vi "Test U8 Logic.vi"() -> ()   [LabVIEW 2021]
uses:
  Source/Abs_Types/U8 Integer/Simple Read.vi
  Source/Constants/Support/U8/Const_U8.lvclass
  C:/TSA/LV_Abstract/Source/Abs_Types/U8 Integer/Abs_U8 Integer.lvclass
  C:/TSA/LV_Abstract/Source/Abs_Types/Integer/Abs_Integer.lvclass
  Source/Constants/Support/U8/U8.vi
  Source/Functions/Logic/Support/NOT/U8/Method.vi
  Source/Functions/Logic/Support/EXOR/U8/Method.vi
  Source/Functions/Logic/Support/EXNOR/U8/Method.vi
  Source/Functions/Logic/Support/NOR/U8/Method.vi
  Source/Functions/Logic/Support/OR/U8/Method.vi
  Source/Functions/Logic/Support/AND/U8/Method.vi
  Source/Abs_Types/U8 Integer/Abs_U8 Integer.lvclass
  C:/Program Files (x86)/National Instruments/LabVIEW 2021/vi.lib/TSA/Abstract Data Classes/Abs_Types/Numeric/Abs_Numeric.lvclass
  C:/Program Files (x86)/National Instruments/LabVIEW 2021/vi.lib/TSA/Abstract Data Classes/Abs_Types/Value/Abs_Value.lvclass
  C:/Program Files (x86)/National Instruments/LabVIEW 2021/vi.lib/TSA/Abstract Data Classes/Abs_Types/Type/Abs_Type.lvclass
  C:/TSA/LV_Abstract/Source/Constants/Support/U8/Const_U8.lvclass
  Source/Functions/Logic/Support/NOT/U8/NOT_U8.lvclass
  Source/Functions/Logic/Support/AND/U8/AND_U8.lvclass
  Source/Functions/Logic/Support/OR/U8/OR_U8.lvclass
  Source/Functions/Logic/Support/NOR/U8/NOR_U8.lvclass
  Source/Functions/Logic/Support/EXNOR/U8/EXNOR_U8.lvclass
  Source/Functions/Logic/Support/EXOR/U8/EXOR_U8.lvclass
panel:
  out "EXNOR":u8 format="%08b"
  out "NOR":u8 format="%08b"
  out "OR":u8 format="%08b"
  out "AND":u8 format="%08b"
  out "EXOR":u8 format="%08b"
  in  "Numeric 2":u8 format="%08b"
  in  "Numeric":u8 format="%08b"
  out "Not":u8 format="%08b"
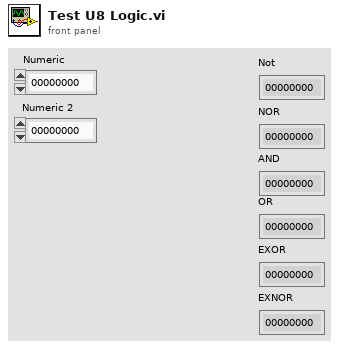
[diagram p1: front panel]
types:
  T1 = typedef "NOT_U8.lvclass/Abs_Type.ctl" = refnum<class "Abs_U8 Integer.lvclass">
  T2 = typedef "EXNOR_U8.lvclass/Abs_Type.ctl" = refnum<class "Abs_U8 Integer.lvclass">
  T3 = typedef "EXOR_U8.lvclass/Abs_Type.ctl" = refnum<class "Abs_U8 Integer.lvclass">
  T4 = typedef "NOR_U8.lvclass/Abs_Type.ctl" = refnum<class "Abs_U8 Integer.lvclass">
  T5 = typedef "OR_U8.lvclass/Abs_Type.ctl" = refnum<class "Abs_U8 Integer.lvclass">
  T6 = typedef "AND_U8.lvclass/Abs_Type.ctl" = refnum<class "Abs_U8 Integer.lvclass">
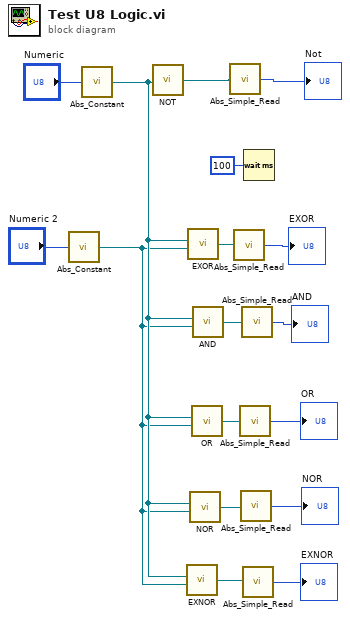
[diagram p0: block diagram]
diagram:
  n1 = call-poly "Abs_Constant.vi"("Value"="Numeric 2") -> ("Constant"=w15:refnum<class "Const_U8.lvclass">)  [unwired: 4 in]
  n2 = call-poly "Abs_Constant.vi"("Value"="Numeric") -> ("Constant"=w16:refnum<class "Const_U8.lvclass">)  [unwired: 4 in]
  n3 = call-poly "NOT.vi"("Bool"=w16) -> ("Result"=w12:T1)  [unwired: 4 in]
  n4 = call-poly "EXNOR.vi"("B"=w15, "A"=w16) -> ("Result"=w5:T2)  [unwired: 4 in]
  n5 = call-poly "EXOR.vi"("B"=w15, "A"=w16) -> ("Result"=w10:T3)  [unwired: 4 in]
  n6 = call-poly "NOR.vi"("B"=w15, "A"=w16) -> ("Result"=w6:T4)  [unwired: 4 in]
  n7 = call-poly "OR.vi"("B"=w15, "A"=w16) -> ("Result"=w7:T5)  [unwired: 4 in]
  n8 = call-poly "AND.vi"("B"=w15, "A"=w16) -> ("Result"=w8:T6)  [unwired: 4 in]
  n9 = call-poly "Abs_Simple_Read.vi"("Read"=w12) -> ("Value"=→"Not":u8)  [unwired: 4 in]
  n10 = call-poly "Abs_Simple_Read.vi"("Read"=w10) -> ("Value"=→"EXOR":u8)  [unwired: 4 in]
  n11 = call-poly "Abs_Simple_Read.vi"("Read"=w7) -> ("Value"=→"OR":u8)  [unwired: 4 in]
  n12 = call-poly "Abs_Simple_Read.vi"("Read"=w6) -> ("Value"=→"NOR":u8)  [unwired: 4 in]
  n13 = call-poly "Abs_Simple_Read.vi"("Read"=w8) -> ("Value"=→"AND":u8)  [unwired: 4 in]
  n14 = call-poly "Abs_Simple_Read.vi"("Read"=w5) -> ("Value"=→"EXNOR":u8)  [unwired: 4 in]
  n15 = Wait (ms)(milliseconds to wait=u32 100) -> ()  [unwired: 1 out]
